vi "start.vi"(8 "error in (no error)":errorcluster, 11 "FPGAWrapperMH120124RAPS_PXI7813R in":refnum<class "FPGAWrapperMH120124RAPS_PXI7813R.lvclass">) -> (0 "error out":errorcluster, 3 "FPGAWrapperMH120124RAPS_PXI7813R out":refnum<class "FPGAWrapperMH120124RAPS_PXI7813R.lvclass">)   [LabVIEW 2010, in "FPGAWrapperMH120124RAPS_PXI7813R.lvclass"]
uses:
  FPGAWrapperMH120124RAPS_PXI7813R.lvclass
  grabber/command_enum.ctl
  class_data.vi
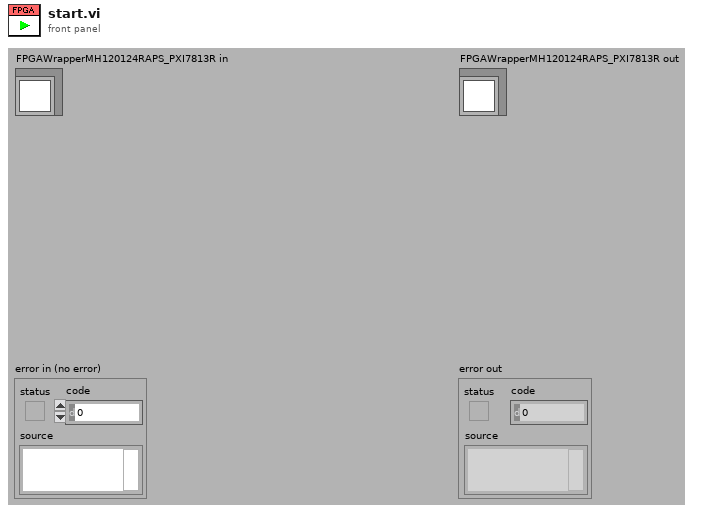
[diagram p1: front panel]
types:
  T1 = typedef "command_enum.ctl" = enum8{"NULL", "update", "start", "stop", "reset", "shut-down"}
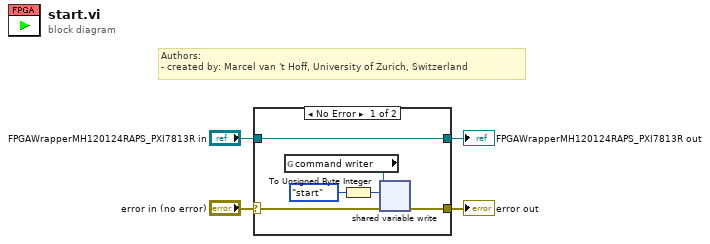
[diagram p0: block diagram]
diagram:
  # "Authors: \n- created by: Marcel van 't Hoff, University of Zurich, Switzerland"
  n1 = case shown="No Error" "error in (no error)" {
    selector: "error in (no error)" -> [w8 w12]
    tunnel: [w7 w12] -> w2
    tunnel: [w10 w11] -> w1
    tunnel: "FPGAWrapperMH120124RAPS_PXI7813R in" -> [w10 w11]
    frame No Error {
      n2 = global read "class_data.vi" "command writer"() -> (w5:refnum<k21>)
      n3 = To Unsigned Byte Integer(number=command_enum."start" ("command")) -> (unsigned 8bit integer=w6:u8)
      n4 = shared-variable-write(w5, w8, w6) -> (w7:errorcluster)  [unwired: 1 in, 2 out]
    }
    frame Error {
    }
  }
  "error out" <- w2
  "FPGAWrapperMH120124RAPS_PXI7813R out" <- w1
